vi "write cal. data.vi"() -> (3 "Success":bool)   [LabVIEW 2018]
uses:
  <vilib>/Utility/file.llb/Read Delimited Spreadsheet (string).vi
  Dll1_x64_191014_0/Dll1_x64_191014_0.lvlib
panel:
  out "status":string
  out "progress":dbl(slide) scale=0.0..100.0
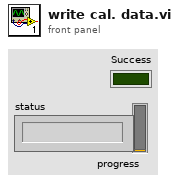
[diagram p1: front panel]
types:
  T1 = enum32{"invalid app kind", "Development System", "Run Time System", "Student Edition", "Embedded LabVIEW", "Evaluation", "Custom"}
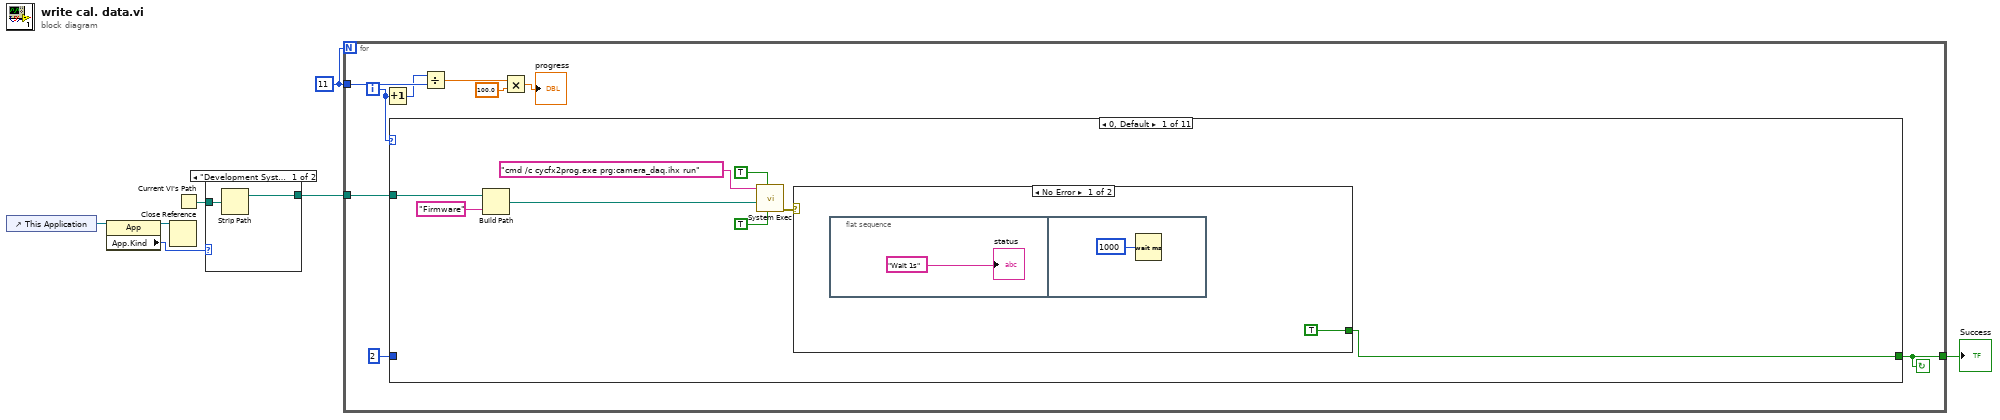
[diagram p0: block diagram]
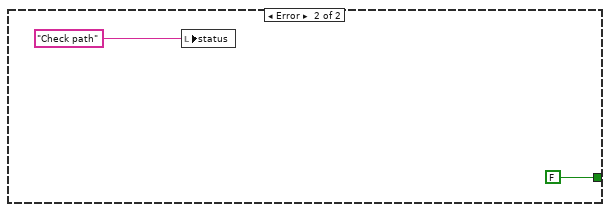
[diagram p2: hidden frame]
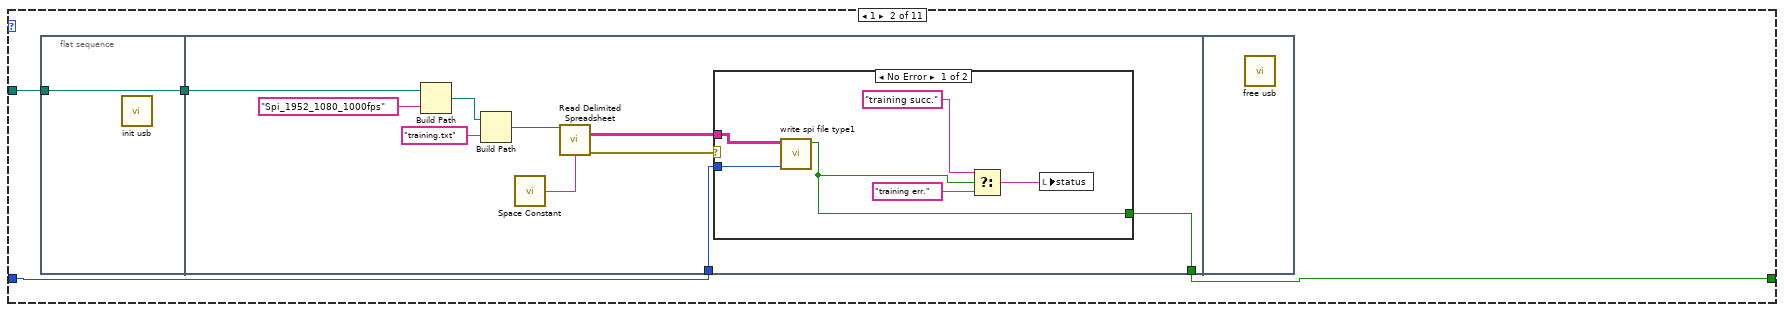
[diagram p3: hidden frame]
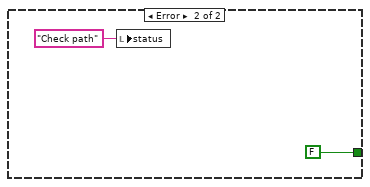
[diagram p4: hidden frame]
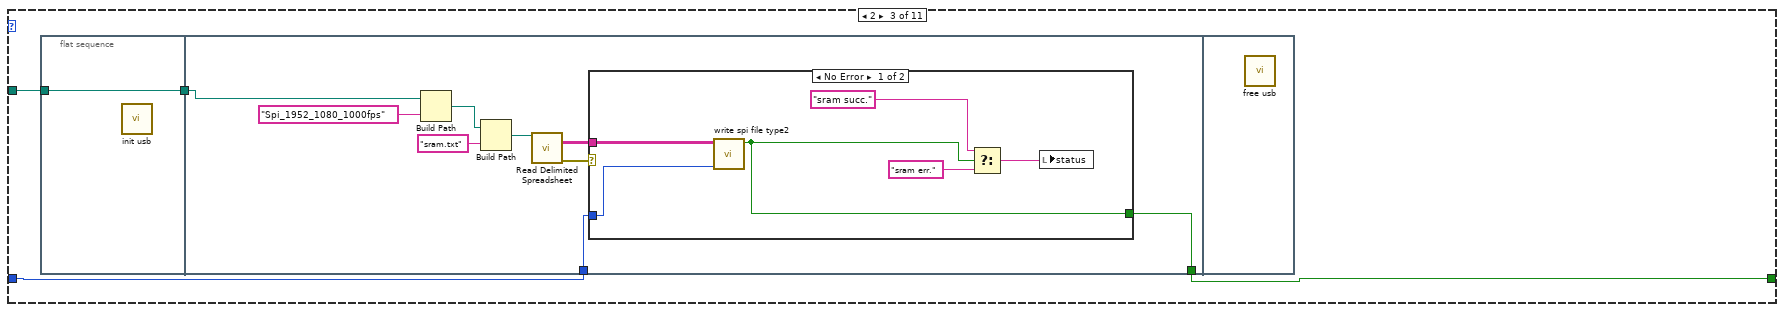
[diagram p5: hidden frame]
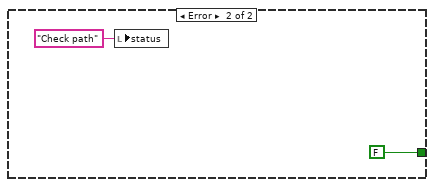
[diagram p6: hidden frame]
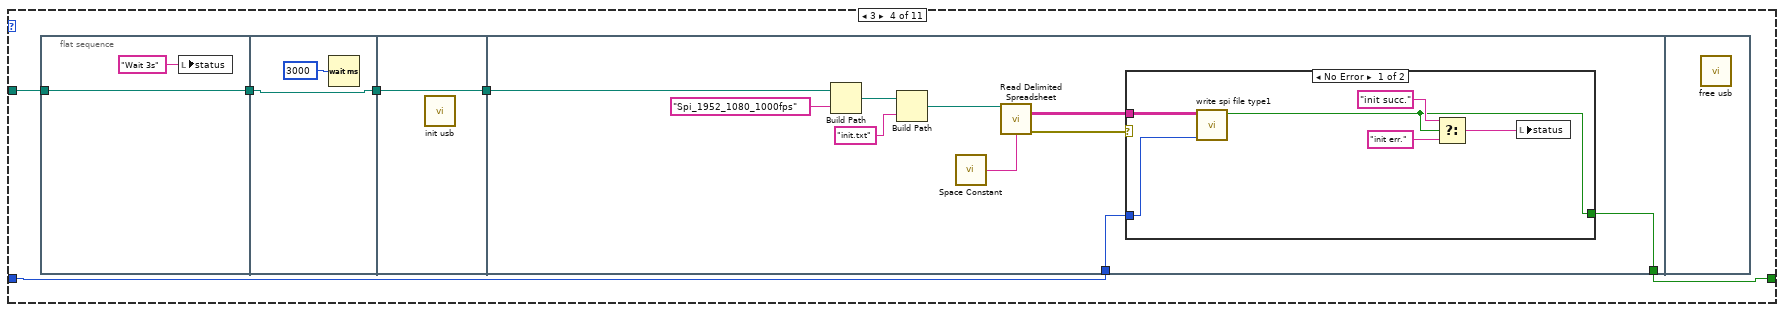
[diagram p7: hidden frame]
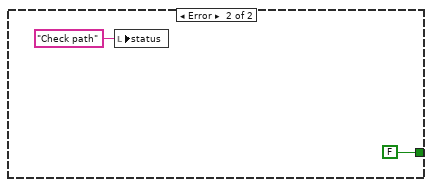
[diagram p8: hidden frame]
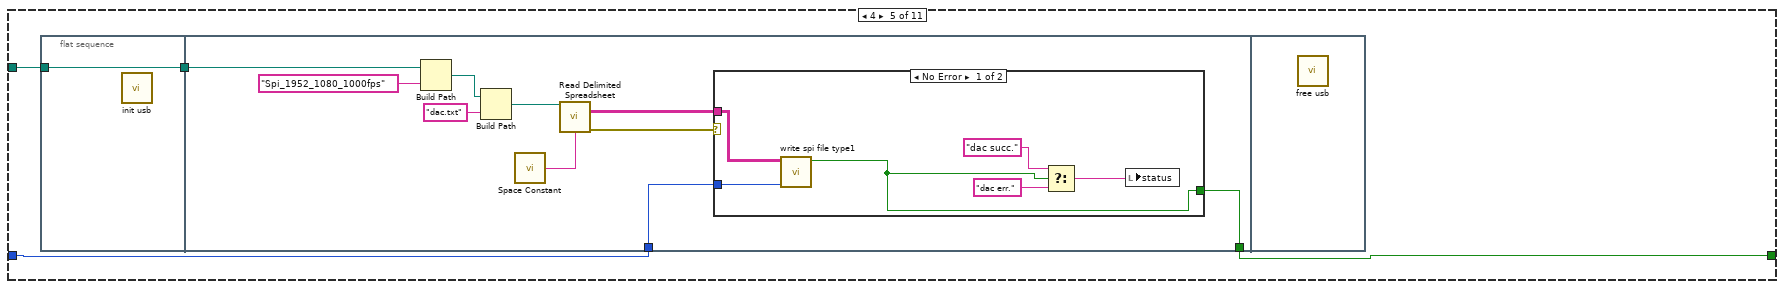
[diagram p9: hidden frame]
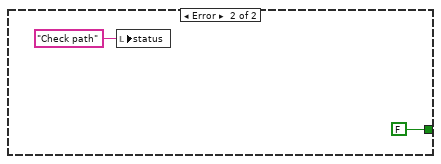
[diagram p10: hidden frame]
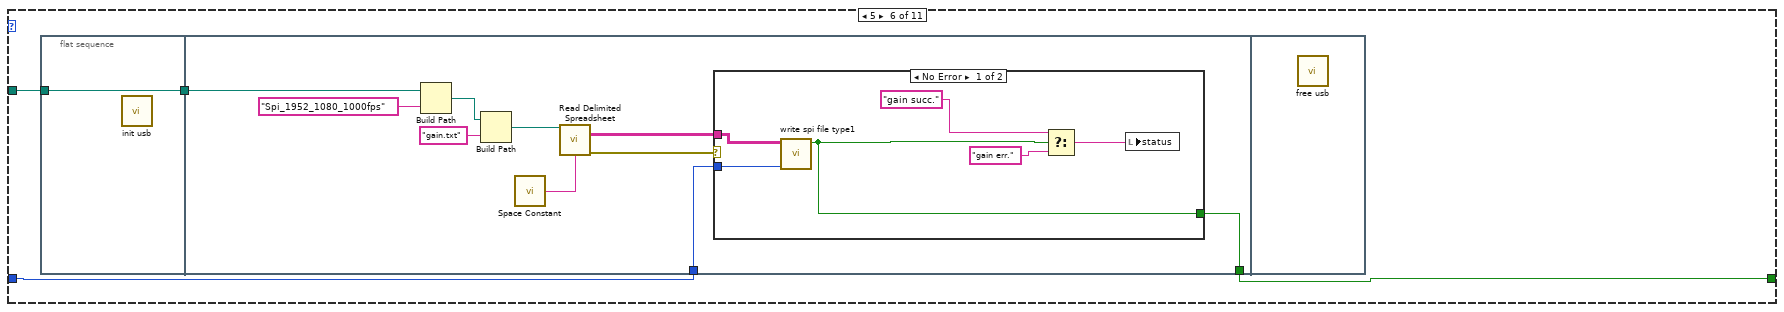
[diagram p11: hidden frame]
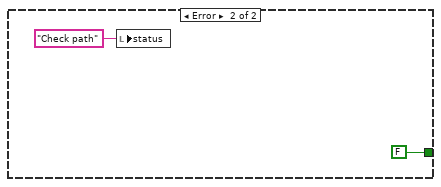
[diagram p12: hidden frame]
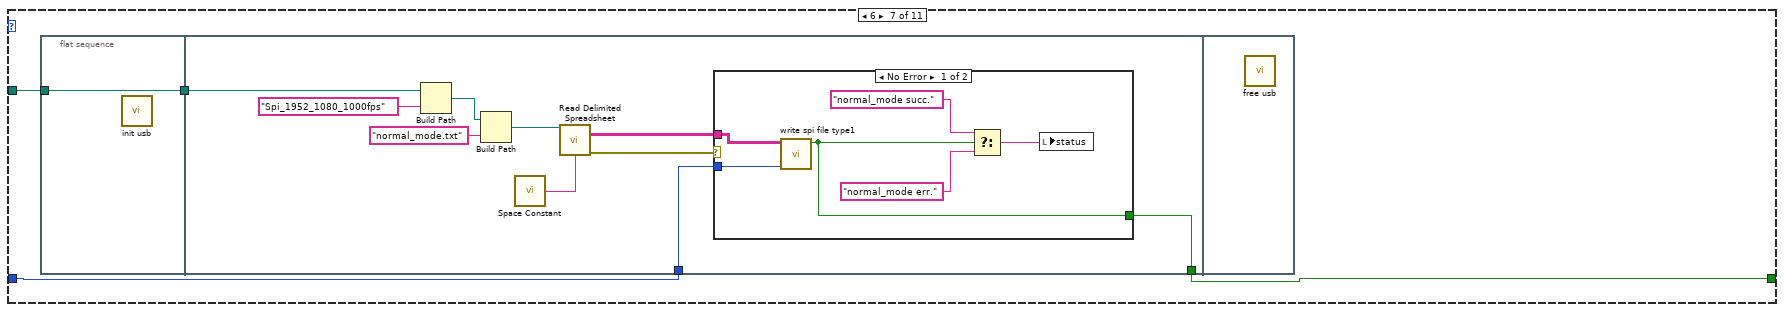
[diagram p13: hidden frame]
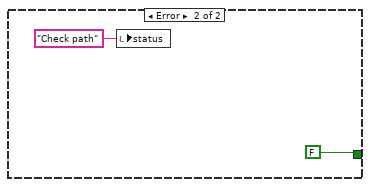
[diagram p14: hidden frame]
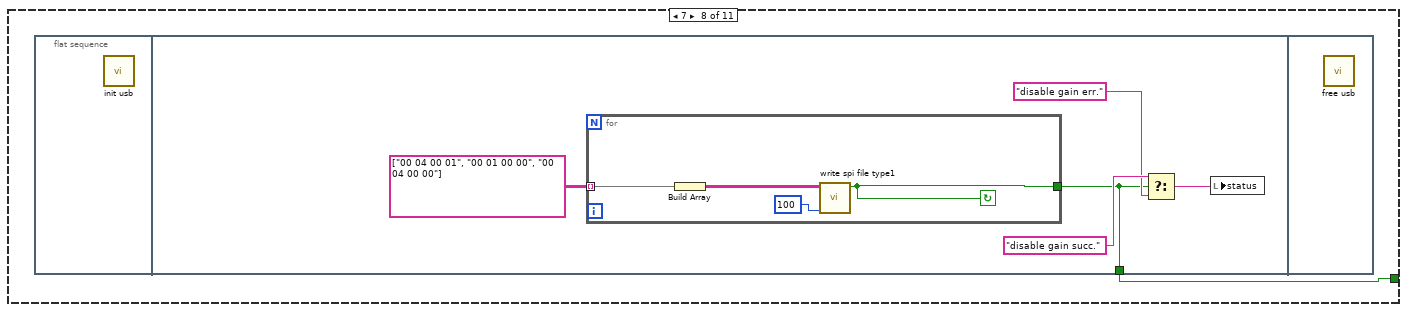
[diagram p15: hidden frame]
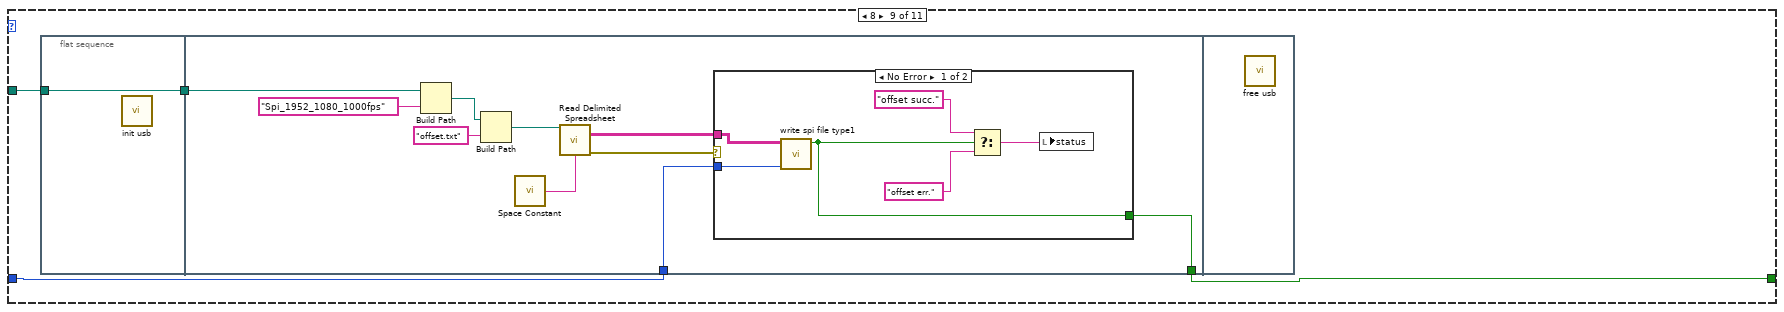
[diagram p16: hidden frame]
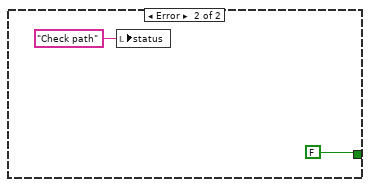
[diagram p17: hidden frame]
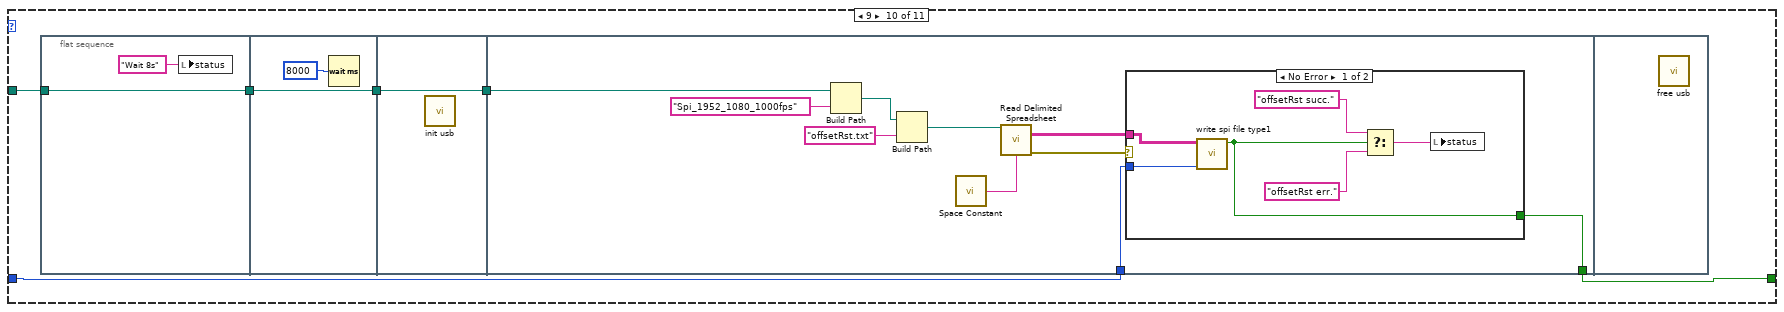
[diagram p18: hidden frame]
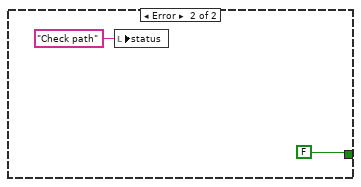
[diagram p19: hidden frame]
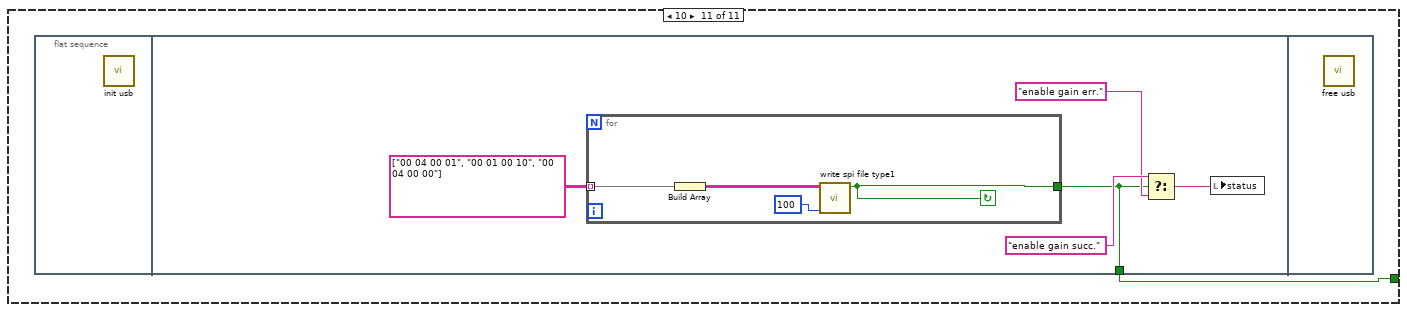
[diagram p20: hidden frame]
diagram:
  w2 = 11
  n1 = control-ref of="This Application"() -> (w4:refnum<vi>)
  n2 = property class="App"(reference=w4) -> (reference out=w5:refnum<vi>, "App.Kind"=w6:T1)  [unwired: 1 in, 1 out]
  n3 = Close Reference(reference=w5) -> ()  [unwired: 1 in, 1 out]
  n4 = Current VI's Path() -> (path=w7:path)
  n5 = case shown="\"Development System\", Default" w6 {
    tunnel: w7 -> [w9 w12]
    tunnel: [w8 w10] -> w3
    frame "Development System", Default {
      n6 = Strip Path(path=w9) -> (stripped path=w8:path)  [unwired: 1 out]
    }
    frame "Run Time System" {
      n7 = Strip Path(path=w12) -> (stripped path=w11:path)  [unwired: 1 out]
      n8 = Strip Path(path=w11) -> (stripped path=w10:path)  [unwired: 1 out]
    }
  }
  n9 = for {
    N: w2 -> [_]
    tunnel: w3 -> [w21]
    tunnel: [w20] -> w1
    tunnel: w2 -> [w18]
    i -> [w19]
    stop <- w20 continue-if-true
    n10 = Increment(x=w19) -> (x+1=w17:i32)
    n11 = case shown="0, Default" w19 {
      tunnel: w21 -> [w24 w38 w60 w82 w111 w134 w157 _ w190 w212 _]
      tunnel: [w23 w35 w59 w81 w110 w133 w156 w178 w189 w213 w240] -> w20
      tunnel: u32 2 ("milliseconds to wait") -> [_ w37 w58 w80 w109 w132 w155 _ w188 w211 _]
      frame 0, Default {
        n12 = Build Path(base path=w24, name or relative path="Firmware") -> (appended path=w26:path)
        n13 = call <vilib>:"System Exec.vi"("run minimized? (F)"=TRUE, "wait until completion? (T)"=TRUE, "working directory"=w26, "command line"="cmd /c cycfx2prog.exe prg:camera_daq.ihx run") -> ("error out"=w22:errorcluster)  [unwired: 4 in, 3 out]
        n14 = case shown="No Error" w22 {
          tunnel: [TRUE ("wait until completion? (T)") FALSE ("wait until completion? (T)")] -> w23
          frame No Error {
            n15 = flat-sequence {
              frame #0 {
                "status" <- "Wait 1s" ("test status")
              }
              frame #1 {
                n16 = Wait (ms)(milliseconds to wait=u32 1000) -> ()  [unwired: 1 out]
              }
            }
          }
          frame Error {
            n17 = local write "status"("Check path" ("status")) -> ()
          }
        }
      }
      frame 1 {
        n18 = flat-sequence {
          tunnel: w38 -> [w39]
          tunnel: [w39] -> w36
          tunnel: w36 -> [w49]
          tunnel: [w42] -> w35
          tunnel: w37 -> [w41]
          frame #0 {
            n19 = call "init usb.vi"() -> ()  [unwired: 12 in]
          }
          frame #1 {
            n20 = Build Path(base path=w49, name or relative path="Spi_1952_1080_1000fps") -> (appended path=w46:path)
            n21 = Build Path(base path=w46, name or relative path="training.txt") -> (appended path=w45:path)
            n22 = call <vilib>:"Space Constant.vi"() -> ("String"=w44:string)
            n23 = call-poly <vilib>:"Read Delimited Spreadsheet.vi"("file path (dialog if empty)"=w45, "delimiter (\\t)"=w44) -> ("all rows"=w43:string[][], "error out"=w40:errorcluster)  [unwired: 8 in, 4 out]
            n24 = case shown="No Error" w40 {
              tunnel: w43 -> [w55 _]
              tunnel: [w53 FALSE ("res")] -> w42
              tunnel: w41 -> [w54 _]
              frame No Error {
                n25 = call "write spi file type1.vi"("milliseconds to wait"=w54, "addr/data"=w55) -> ("res"=w53:bool)  [unwired: 9 in]
                n26 = Select(t="training succ." ("status"), s=w53, f="training err.") -> (s? t:f=w52:string)
                n27 = local write "status"(w52) -> ()
              }
              frame Error {
                n28 = local write "status"("Check path" ("status")) -> ()
              }
            }
          }
          frame #2 {
            n29 = call "free usb.vi"() -> ()  [unwired: 12 in]
          }
        }
      }
      frame 2 {
        n30 = flat-sequence {
          tunnel: w60 -> [w62]
          tunnel: [w62] -> w61
          tunnel: w61 -> [w70]
          tunnel: [w65] -> w59
          tunnel: w58 -> [w64]
          frame #0 {
            n31 = call "init usb.vi"() -> ()  [unwired: 12 in]
          }
          frame #1 {
            n32 = Build Path(base path=w70, name or relative path="Spi_1952_1080_1000fps") -> (appended path=w68:path)
            n33 = Build Path(base path=w68, name or relative path="sram.txt") -> (appended path=w67:path)
            n34 = call-poly <vilib>:"Read Delimited Spreadsheet.vi"("file path (dialog if empty)"=w67) -> ("all rows"=w66:string[][], "error out"=w63:errorcluster)  [unwired: 9 in, 4 out]
            n35 = case shown="No Error" w63 {
              tunnel: w66 -> [w77 _]
              tunnel: [w72 FALSE ("res")] -> w65
              tunnel: w64 -> [w76 _]
              frame No Error {
                n36 = call "write spi file type2.vi"("milliseconds to wait"=w76, "addr/data"=w77) -> ("res"=w72:bool)  [unwired: 9 in]
                n37 = Select(t="sram succ." ("status"), s=w72, f="sram err.") -> (s? t:f=w75:string)
                n38 = local write "status"(w75) -> ()
              }
              frame Error {
                n39 = local write "status"("Check path" ("status")) -> ()
              }
            }
          }
          frame #2 {
            n40 = call "free usb.vi"() -> ()  [unwired: 12 in]
          }
        }
      }
      frame 3 {
        n41 = flat-sequence {
          tunnel: w82 -> [w87]
          tunnel: [w87] -> w85
          tunnel: [w89] -> w84
          tunnel: w85 -> [w89]
          tunnel: w84 -> [w90]
          tunnel: [w90] -> w83
          tunnel: w83 -> [w99]
          tunnel: [w93] -> w81
          tunnel: w80 -> [w92]
          frame #0 {
            n42 = local write "status"("Wait 3s" ("result")) -> ()
          }
          frame #1 {
            n43 = Wait (ms)(milliseconds to wait=u32 3000) -> ()  [unwired: 1 out]
          }
          frame #2 {
            n44 = call "init usb.vi"() -> ()  [unwired: 12 in]
          }
          frame #3 {
            n45 = Build Path(base path=w99, name or relative path="Spi_1952_1080_1000fps") -> (appended path=w97:path)
            n46 = Build Path(base path=w97, name or relative path="init.txt") -> (appended path=w96:path)
            n47 = call <vilib>:"Space Constant.vi"() -> ("String"=w95:string)
            n48 = call-poly <vilib>:"Read Delimited Spreadsheet.vi"("file path (dialog if empty)"=w96, "delimiter (\\t)"=w95) -> ("all rows"=w94:string[][], "error out"=w91:errorcluster)  [unwired: 8 in, 4 out]
            n49 = case shown="No Error" w91 {
              tunnel: w94 -> [w106 _]
              tunnel: [w101 FALSE ("res")] -> w93
              tunnel: w92 -> [w105 _]
              frame No Error {
                n50 = call "write spi file type1.vi"("milliseconds to wait"=w105, "addr/data"=w106) -> ("res"=w101:bool)  [unwired: 9 in]
                n51 = Select(t="init succ." ("status"), s=w101, f="init err.") -> (s? t:f=w104:string)
                n52 = local write "status"(w104) -> ()
              }
              frame Error {
                n53 = local write "status"("Check path" ("status")) -> ()
              }
            }
          }
          frame #4 {
            n54 = call "free usb.vi"() -> ()  [unwired: 12 in]
          }
        }
      }
      frame 4 {
        n55 = flat-sequence {
          tunnel: w111 -> [w113]
          tunnel: [w113] -> w112
          tunnel: w112 -> [w122]
          tunnel: [w115] -> w110
          tunnel: w109 -> [w116]
          frame #0 {
            n56 = call "init usb.vi"() -> ()  [unwired: 12 in]
          }
          frame #1 {
            n57 = Build Path(base path=w122, name or relative path="Spi_1952_1080_1000fps") -> (appended path=w120:path)
            n58 = Build Path(base path=w120, name or relative path="dac.txt") -> (appended path=w119:path)
            n59 = call <vilib>:"Space Constant.vi"() -> ("String"=w118:string)
            n60 = call-poly <vilib>:"Read Delimited Spreadsheet.vi"("file path (dialog if empty)"=w119, "delimiter (\\t)"=w118) -> ("all rows"=w117:string[][], "error out"=w114:errorcluster)  [unwired: 8 in, 4 out]
            n61 = case shown="No Error" w114 {
              tunnel: w117 -> [w129 _]
              tunnel: w116 -> [w128 _]
              tunnel: [w124 FALSE ("res")] -> w115
              frame No Error {
                n62 = call "write spi file type1.vi"("milliseconds to wait"=w128, "addr/data"=w129) -> ("res"=w124:bool)  [unwired: 9 in]
                n63 = Select(t="dac succ." ("status"), s=w124, f="dac err.") -> (s? t:f=w127:string)
                n64 = local write "status"(w127) -> ()
              }
              frame Error {
                n65 = local write "status"("Check path" ("status")) -> ()
              }
            }
          }
          frame #2 {
            n66 = call "free usb.vi"() -> ()  [unwired: 12 in]
          }
        }
      }
      frame 5 {
        n67 = flat-sequence {
          tunnel: w134 -> [w136]
          tunnel: [w136] -> w135
          tunnel: w135 -> [w145]
          tunnel: [w139] -> w133
          tunnel: w132 -> [w138]
          frame #0 {
            n68 = call "init usb.vi"() -> ()  [unwired: 12 in]
          }
          frame #1 {
            n69 = Build Path(base path=w145, name or relative path="Spi_1952_1080_1000fps") -> (appended path=w143:path)
            n70 = Build Path(base path=w143, name or relative path="gain.txt") -> (appended path=w142:path)
            n71 = call <vilib>:"Space Constant.vi"() -> ("String"=w141:string)
            n72 = call-poly <vilib>:"Read Delimited Spreadsheet.vi"("file path (dialog if empty)"=w142, "delimiter (\\t)"=w141) -> ("all rows"=w140:string[][], "error out"=w137:errorcluster)  [unwired: 8 in, 4 out]
            n73 = case shown="No Error" w137 {
              tunnel: w140 -> [w152 _]
              tunnel: [w147 FALSE ("res")] -> w139
              tunnel: w138 -> [w151 _]
              frame No Error {
                n74 = call "write spi file type1.vi"("milliseconds to wait"=w151, "addr/data"=w152) -> ("res"=w147:bool)  [unwired: 9 in]
                n75 = Select(t="gain succ." ("status"), s=w147, f="gain err.") -> (s? t:f=w150:string)
                n76 = local write "status"(w150) -> ()
              }
              frame Error {
                n77 = local write "status"("Check path" ("status")) -> ()
              }
            }
          }
          frame #2 {
            n78 = call "free usb.vi"() -> ()  [unwired: 12 in]
          }
        }
      }
      frame 6 {
        n79 = flat-sequence {
          tunnel: w157 -> [w159]
          tunnel: [w159] -> w158
          tunnel: w158 -> [w168]
          tunnel: [w162] -> w156
          tunnel: w155 -> [w161]
          frame #0 {
            n80 = call "init usb.vi"() -> ()  [unwired: 12 in]
          }
          frame #1 {
            n81 = Build Path(base path=w168, name or relative path="Spi_1952_1080_1000fps") -> (appended path=w166:path)
            n82 = Build Path(base path=w166, name or relative path="normal_mode.txt") -> (appended path=w165:path)
            n83 = call <vilib>:"Space Constant.vi"() -> ("String"=w164:string)
            n84 = call-poly <vilib>:"Read Delimited Spreadsheet.vi"("file path (dialog if empty)"=w165, "delimiter (\\t)"=w164) -> ("all rows"=w163:string[][], "error out"=w160:errorcluster)  [unwired: 8 in, 4 out]
            n85 = case shown="No Error" w160 {
              tunnel: w163 -> [w175 _]
              tunnel: [w170 FALSE ("res")] -> w162
              tunnel: w161 -> [w174 _]
              frame No Error {
                n86 = call "write spi file type1.vi"("milliseconds to wait"=w174, "addr/data"=w175) -> ("res"=w170:bool)  [unwired: 9 in]
                n87 = Select(t="normal_mode succ." ("status"), s=w170, f="normal_mode err.") -> (s? t:f=w173:string)
                n88 = local write "status"(w173) -> ()
              }
              frame Error {
                n89 = local write "status"("Check path" ("status")) -> ()
              }
            }
          }
          frame #2 {
            n90 = call "free usb.vi"() -> ()  [unwired: 12 in]
          }
        }
      }
      frame 7 {
        n91 = flat-sequence {
          tunnel: [w179] -> w178
          frame #0 {
            n92 = call "init usb.vi"() -> ()  [unwired: 12 in]
          }
          frame #1 {
            n93 = for {
              tunnel: string[][] [["00 04 00 01"], ["00 01 00 00"], ["00 04 00 00"]] ("all rows") -> [w187] mode=indexing
              tunnel: [w185] -> w179
              stop <- w185 continue-if-true
              n94 = Build Array(w187) -> (w186:string[][])
              n95 = call "write spi file type1.vi"("milliseconds to wait"=u32 100, "addr/data"=w186) -> ("res"=w185:bool)  [unwired: 9 in]
            }
            n96 = Select(t="disable gain succ." ("status"), s=w179, f="disable gain err.") -> (s? t:f=w182:string)
            n97 = local write "status"(w182) -> ()
          }
          frame #2 {
            n98 = call "free usb.vi"() -> ()  [unwired: 12 in]
          }
        }
      }
      frame 8 {
        n99 = flat-sequence {
          tunnel: w190 -> [w192]
          tunnel: [w192] -> w191
          tunnel: w191 -> [w201]
          tunnel: [w195] -> w189
          tunnel: w188 -> [w194]
          frame #0 {
            n100 = call "init usb.vi"() -> ()  [unwired: 12 in]
          }
          frame #1 {
            n101 = Build Path(base path=w201, name or relative path="Spi_1952_1080_1000fps") -> (appended path=w199:path)
            n102 = Build Path(base path=w199, name or relative path="offset.txt") -> (appended path=w198:path)
            n103 = call <vilib>:"Space Constant.vi"() -> ("String"=w197:string)
            n104 = call-poly <vilib>:"Read Delimited Spreadsheet.vi"("file path (dialog if empty)"=w198, "delimiter (\\t)"=w197) -> ("all rows"=w196:string[][], "error out"=w193:errorcluster)  [unwired: 8 in, 4 out]
            n105 = case shown="No Error" w193 {
              tunnel: w196 -> [w208 _]
              tunnel: [w203 FALSE ("res")] -> w195
              tunnel: w194 -> [w207 _]
              frame No Error {
                n106 = call "write spi file type1.vi"("milliseconds to wait"=w207, "addr/data"=w208) -> ("res"=w203:bool)  [unwired: 9 in]
                n107 = Select(t="offset succ." ("status"), s=w203, f="offset err.") -> (s? t:f=w206:string)
                n108 = local write "status"(w206) -> ()
              }
              frame Error {
                n109 = local write "status"("Check path" ("status")) -> ()
              }
            }
          }
          frame #2 {
            n110 = call "free usb.vi"() -> ()  [unwired: 12 in]
          }
        }
      }
      frame 9 {
        n111 = flat-sequence {
          tunnel: w212 -> [w218]
          tunnel: [w218] -> w216
          tunnel: [w220] -> w215
          tunnel: w216 -> [w220]
          tunnel: [w221] -> w214
          tunnel: w215 -> [w221]
          tunnel: w214 -> [w230]
          tunnel: [w224] -> w213
          tunnel: w211 -> [w223]
          frame #0 {
            n112 = local write "status"("Wait 8s" ("result")) -> ()
          }
          frame #1 {
            n113 = Wait (ms)(milliseconds to wait=u32 8000) -> ()  [unwired: 1 out]
          }
          frame #2 {
            n114 = call "init usb.vi"() -> ()  [unwired: 12 in]
          }
          frame #3 {
            n115 = Build Path(base path=w230, name or relative path="Spi_1952_1080_1000fps") -> (appended path=w228:path)
            n116 = Build Path(base path=w228, name or relative path="offsetRst.txt") -> (appended path=w227:path)
            n117 = call <vilib>:"Space Constant.vi"() -> ("String"=w226:string)
            n118 = call-poly <vilib>:"Read Delimited Spreadsheet.vi"("file path (dialog if empty)"=w227, "delimiter (\\t)"=w226) -> ("all rows"=w225:string[][], "error out"=w222:errorcluster)  [unwired: 8 in, 4 out]
            n119 = case shown="No Error" w222 {
              tunnel: w225 -> [w237 _]
              tunnel: [w232 FALSE ("res")] -> w224
              tunnel: w223 -> [w236 _]
              frame No Error {
                n120 = call "write spi file type1.vi"("milliseconds to wait"=w236, "addr/data"=w237) -> ("res"=w232:bool)  [unwired: 9 in]
                n121 = Select(t="offsetRst succ." ("status"), s=w232, f="offsetRst err.") -> (s? t:f=w235:string)
                n122 = local write "status"(w235) -> ()
              }
              frame Error {
                n123 = local write "status"("Check path" ("status")) -> ()
              }
            }
          }
          frame #4 {
            n124 = call "free usb.vi"() -> ()  [unwired: 12 in]
          }
        }
      }
      frame 10 {
        n125 = flat-sequence {
          tunnel: [w241] -> w240
          frame #0 {
            n126 = call "init usb.vi"() -> ()  [unwired: 12 in]
          }
          frame #1 {
            n127 = for {
              tunnel: string[][] [["00 04 00 01"], ["00 01 00 10"], ["00 04 00 00"]] ("all rows") -> [w249] mode=indexing
              tunnel: [w247] -> w241
              stop <- w247 continue-if-true
              n128 = Build Array(w249) -> (w248:string[][])
              n129 = call "write spi file type1.vi"("milliseconds to wait"=u32 100, "addr/data"=w248) -> ("res"=w247:bool)  [unwired: 9 in]
            }
            n130 = Select(t="enable gain succ." ("status"), s=w241, f="enable gain err.") -> (s? t:f=w244:string)
            n131 = local write "status"(w244) -> ()
          }
          frame #2 {
            n132 = call "free usb.vi"() -> ()  [unwired: 12 in]
          }
        }
      }
    }
    n133 = Divide(x=w17, y=w18) -> (x/y=w16:dbl)
    n134 = Multiply(x=w16, y=100.0) -> (x*y=→"progress":dbl)
  }
  "Success" <- w1
